vi "Test Window Launched.vi"(8 "error in (no error)":errorcluster, 9 "VI Refnum":refnum<vi>, 10 "Window Name":string, 11 "Test in":refnum<class "Test.lvclass">) -> (0 "error out":errorcluster, 3 "Test out":refnum<class "Test.lvclass">)   [LabVIEW 2017, in "Test.lvlib" / "Test.lvclass"]
uses:
  Test.lvclass
  C:/Program Files (x86)/National Instruments/LabVIEW 2017/vi.lib/ActorFramework/Actor/Actor.lvclass
  <vilib>/ActorFramework/Actor/Actor.lvclass/Actor.ctl
  Test.lvclass/Test.ctl
  Test Messages/Test Window Launched Msg/Test Window Launched Msg.lvclass/Test Window Launched Msg.ctl
  <vilib>/ActorFramework/Message Enqueuer/Message Enqueuer.lvclass/Message Enqueuer.ctl
  <vilib>/ActorFramework/Message Enqueuer/Enqueue.vi
  Test Messages/Test Window Launched Msg/Test Window Launched Msg.lvclass
  C:/Program Files (x86)/National Instruments/LabVIEW 2017/vi.lib/ActorFramework/Message/Message.lvclass
  <vilib>/ActorFramework/Message Priority Queue/Priority Enqueue.vi
  <vilib>/ActorFramework/Actor/Actor.lvclass
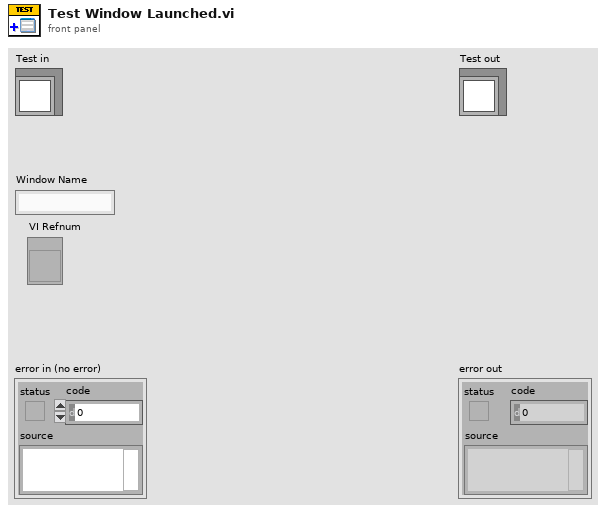
[diagram p1: front panel]
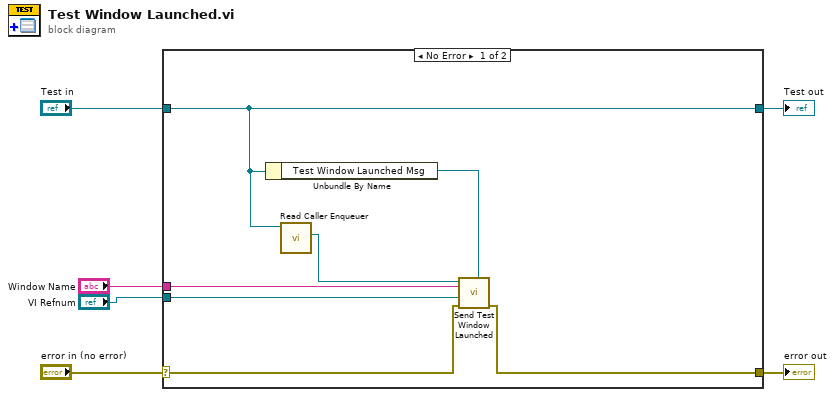
[diagram p0: block diagram]
diagram:
  n1 = case shown="No Error" "error in (no error)" {
    selector: "error in (no error)" -> [w11 w15]
    tunnel: [w10 w15] -> w5
    tunnel: [w13 w14] -> w3
    tunnel: "Test in" -> [w13 w14]
    tunnel: "VI Refnum" -> [w8 _]
    tunnel: "Window Name" -> [w7 _]
    frame No Error {
      n2 = Unbundle By Name(w13) -> ("Test Window Launched Msg"=w9:refnum<class "Test Window Launched Msg.lvclass">)
      n3 = call <vilib>:"Read Caller Enqueuer.vi"("Actor"=w13) -> ("Caller Enqueuer"=w12:refnum<class "Message Enqueuer.lvclass">)  [unwired: 10 in]
      n4 = call "Send Test Window Launched.vi"("Message Type"=w9, "error in (no error)"=w11, "VI Refnum"=w8, "Window Name"=w7, "Message Enqueuer"=w12) -> ("error out"=w10:errorcluster)  [unwired: 5 in, 1 out]
    }
    frame Error {
    }
  }
  "error out" <- w5
  "Test out" <- w3
